vi "Evaluate Analog Edge Trigger.vi"(8 "error in (no error)":errorcluster, 10 "Trigger Data":dbl[](array[numeric]), 11 "Analog Edge Trigger in":refnum<class "Analog Edge Trigger.lvclass">) -> (0 "error out":errorcluster, 2 "Trigger":bool, 3 "Analog Edge Trigger out":refnum<class "Analog Edge Trigger.lvclass">)   [LabVIEW 2012, in "Waveform Data Logger Engine.lvlib" / "Analog Edge Trigger.lvclass"]
uses:
  Analog Edge Trigger.lvclass
  Analog Edge Trigger.lvclass/Analog Edge Trigger.ctl
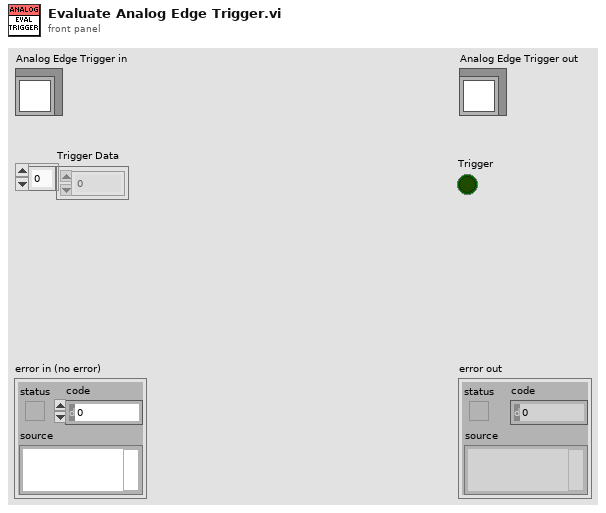
[diagram p1: front panel]
types:
  T1 = typedef "Waveform Data Logger Engine.lvlib/Analog Edge Trigger.lvclass/Analog Slope Type.ctl" = enum16{"Rising", "Falling"}
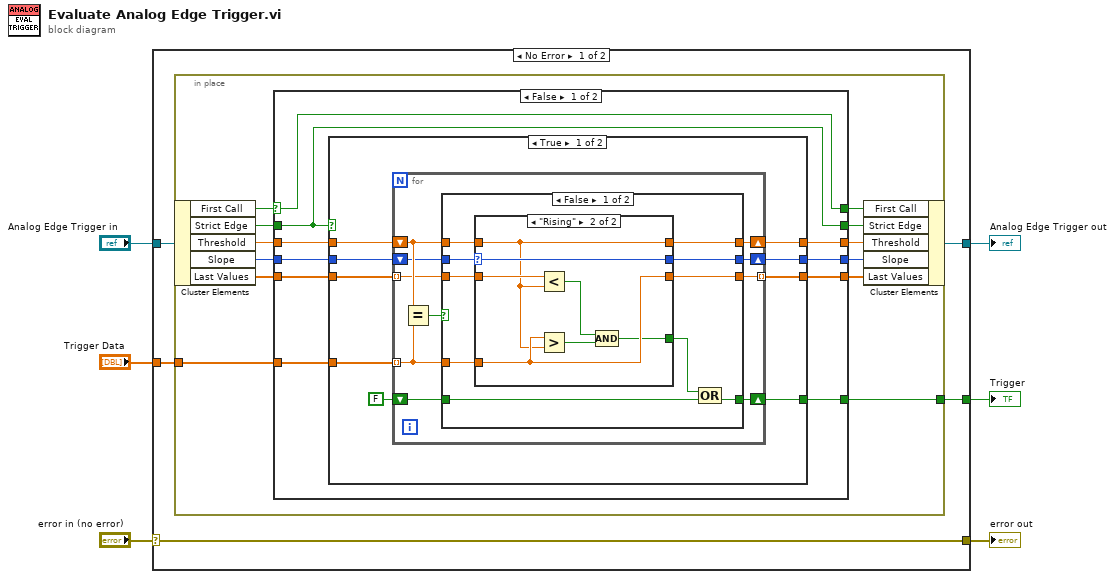
[diagram p0: block diagram]
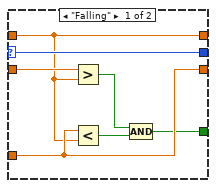
[diagram p2: hidden frame]
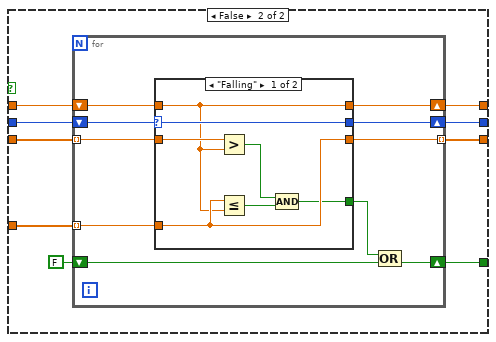
[diagram p4: hidden frame]
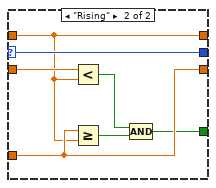
[diagram p5: hidden frame]
diagram:
  n1 = case shown="No Error" "error in (no error)" {
    selector: "error in (no error)" -> [w7 w119]
    tunnel: "Analog Edge Trigger in" -> [w11 w118]
    tunnel: "Trigger Data" -> [w10 _]
    tunnel: [w9 _] -> w4
    tunnel: [w8 w118] -> w3
    tunnel: [w7 w119] -> w1
    frame No Error {
      n2 = in-place {
        in-place-border: w10 -> [w14]
        in-place-border: [w16] -> w9
        n3 = in-place-cluster #1(w11) -> ("First Call"=w17:bool, "Strict Edge"=w13:bool, "Threshold"=w22:dbl, "Slope"=w20:T1, "Last Values"=w19:dbl[])
        n4 = case shown="False" w17 {
          selector: w17 -> [w25 _]
          tunnel: [w33 w117] -> w23
          tunnel: w22 -> [w32 w117]
          tunnel: [w31 w116] -> w21
          tunnel: w20 -> [w30 w116]
          tunnel: w19 -> [w29 _]
          tunnel: [w28 w115] -> w18
          tunnel: [w27 _] -> w16
          tunnel: w14 -> [w26 w115]
          tunnel: [w25 _] -> w15
          tunnel: w13 -> [w24 w114]
          tunnel: [w24 w114] -> w12
          frame False {
            n5 = case shown="True" w24 {
              tunnel: [w42 w89] -> w33
              tunnel: w32 -> [w41 w88]
              tunnel: [w40 w87] -> w31
              tunnel: w30 -> [w39 w86]
              tunnel: w29 -> [w38 w85]
              tunnel: [w37 w84] -> w28
              tunnel: [w36 w83] -> w27
              tunnel: w26 -> [w35 w82]
              frame True {
                n6 = for {
                  tunnel: w38 -> [w47] mode=indexing
                  tunnel: [w46] -> w37 mode=indexing
                  tunnel: w35 -> [w44] mode=indexing
                  shift-right: [w51] -> w42
                  shift-left: w41 -> [w50]
                  shift-right: [w49] -> w40
                  shift-left: w39 -> [w48]
                  shift-right: [w45] -> w36
                  shift-left: FALSE -> [w43]
                  n7 = Equal?(x=w50, y=w44) -> (x = y?=w52:bool)
                  n8 = case shown="False" w52 {
                    tunnel: [w56 w80] -> w51
                    tunnel: w50 -> [w61 w80]
                    tunnel: [w57 w79] -> w49
                    tunnel: w48 -> [w62 w79]
                    tunnel: w47 -> [w60 w78]
                    tunnel: [w58 w78] -> w46
                    tunnel: [w54 w77] -> w45
                    tunnel: w44 -> [w59 _]
                    tunnel: w43 -> [w53 w77]
                    frame False {
                      n9 = case shown="\"Rising\"" w62 {
                        selector: w62 -> [w65 w72]
                        tunnel: w61 -> [w64 w71]
                        tunnel: w60 -> [w69 w76]
                        tunnel: w59 -> [w66 w73]
                        tunnel: [w66 w73] -> w58
                        tunnel: [w65 w72] -> w57
                        tunnel: [w64 w71] -> w56
                        tunnel: [w63 w70] -> w55
                        frame "Falling" {
                          n10 = Greater?(x=w69, y=w64) -> (0:w68:bool)
                          n11 = Less?(x=w66, y=w64) -> (x < y?=w67:bool)
                          n12 = Compound Arithmetic op=AND(w68, w67) -> (w63:bool)
                        }
                        frame "Rising" {
                          n13 = Less?(x=w76, y=w71) -> (x < y?=w75:bool)
                          n14 = Greater?(x=w73, y=w71) -> (0:w74:bool)
                          n15 = Compound Arithmetic op=AND(w75, w74) -> (w70:bool)
                        }
                      }
                      n16 = Compound Arithmetic op=OR(w55, w53) -> (w54:bool)
                    }
                    frame True {
                      # "Do not keep track of values that are exactly equal to the threshold, so that we can tell if a previous value was actually above or below that threshold."
                    }
                  }
                }
              }
              frame False {
                n17 = for {
                  tunnel: w85 -> [w95] mode=indexing
                  tunnel: [w94] -> w84 mode=indexing
                  tunnel: w82 -> [w92] mode=indexing
                  shift-right: [w99] -> w89
                  shift-left: w88 -> [w98]
                  shift-right: [w97] -> w87
                  shift-left: w86 -> [w96]
                  shift-right: [w93] -> w83
                  shift-left: FALSE -> [w91]
                  n18 = case shown="\"Falling\"" w96 {
                    selector: w96 -> [w102 w109]
                    tunnel: w98 -> [w101 w108]
                    tunnel: w95 -> [w106 w113]
                    tunnel: w92 -> [w103 w110]
                    tunnel: [w103 w110] -> w94
                    tunnel: [w102 w109] -> w97
                    tunnel: [w101 w108] -> w99
                    tunnel: [w100 w107] -> w90
                    frame "Falling" {
                      n19 = Greater?(x=w106, y=w101) -> (0:w105:bool)
                      n20 = Less Or Equal?(x=w103, y=w101) -> (x <= y?=w104:bool)
                      n21 = Compound Arithmetic op=AND(w105, w104) -> (w100:bool)
                    }
                    frame "Rising" {
                      n22 = Less?(x=w113, y=w108) -> (x < y?=w112:bool)
                      n23 = Greater Or Equal?(x=w110, y=w108) -> (x >= y?=w111:bool)
                      n24 = Compound Arithmetic op=AND(w112, w111) -> (w107:bool)
                    }
                  }
                  n25 = Compound Arithmetic op=OR(w90, w91) -> (w93:bool)
                }
              }
            }
          }
          frame True {
            # "Just latch the trigger value on the first call. The trigger takes at least two timesteps to trigger."
          }
        }
        n26 = in-place-cluster #1("First Call"=w15, "Strict Edge"=w12, "Threshold"=w23, "Slope"=w21, "Last Values"=w18) -> (w8:refnum<class "Analog Edge Trigger.lvclass">)
      }
    }
    frame Error {
    }
  }
  "error out" <- w1
  "Analog Edge Trigger out" <- w3
  "Trigger" <- w4
